vi "PDCDetectDrop.vi"(6 "Sensitivity [0-100]":dbl, 8 "Error In":errorcluster, 9 "RefImage":u16[](array[numeric]), 10 "CurrentImage":u16[](array[numeric]), 11 "DataDisplay":refnum<queue>) -> (0 "Error Out":errorcluster)   [LabVIEW 2015]
uses:
  TypeDefs/MessageCluster.ctl
  <vilib>/Analysis/NI_AALBase.lvlib
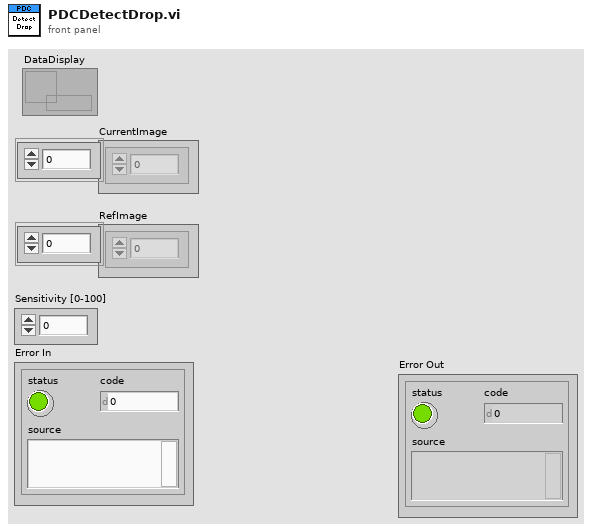
[diagram p1: front panel]
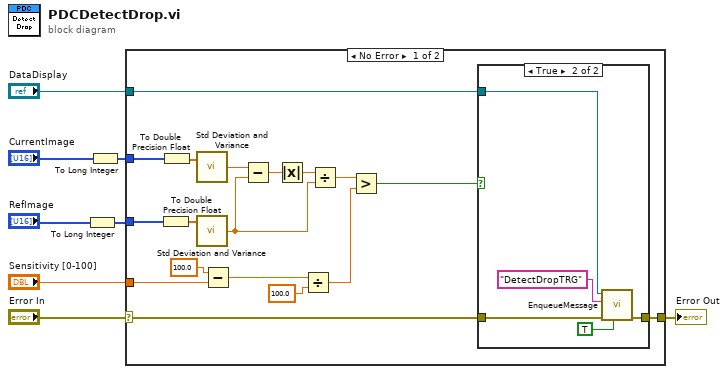
[diagram p0: block diagram]
diagram:
  n1 = To Long Integer(number="RefImage") -> (32bit integer=w4:i32[])
  n2 = To Long Integer(number="CurrentImage") -> (32bit integer=w2:i32[])
  n3 = case shown="No Error" "Error In" {
    selector: "Error In" -> [w25 w33]
    tunnel: [w26 w33] -> w7
    tunnel: "DataDisplay" -> [w24 _]
    tunnel: w4 -> [w22 _]
    tunnel: w2 -> [w23 _]
    tunnel: "Sensitivity [0-100]" -> [w10 _]
    frame No Error {
      n4 = To Double Precision Float(number=w22) -> (double precision float=w20:dbl[])
      n5 = To Double Precision Float(number=w23) -> (double precision float=w19:dbl[])
      n6 = call <vilib>:"Std Deviation and Variance.vi"("X"=w19) -> ("standard deviation"=w17:dbl)  [unwired: 1 in, 2 out]
      n7 = call <vilib>:"Std Deviation and Variance.vi"("X"=w20) -> ("standard deviation"=w14:dbl)  [unwired: 1 in, 2 out]
      n8 = Subtract(x=100.0, y=w10) -> (x-y=w9:dbl)
      n9 = Subtract(x=w17, y=w14) -> (x-y=w18:dbl)
      n10 = Absolute Value(x=w18) -> (abs(x)=w16:dbl)
      n11 = Divide(x=w9, y=100.0) -> (x/y=w11:dbl)
      n12 = Divide(x=w16, y=w14) -> (x/y=w15:dbl)
      n13 = Greater?(x=w15, y=w11) -> (0:w21:bool)
      n14 = case shown="True" w21 {
        tunnel: [w27 w32] -> w26
        tunnel: w25 -> [w27 w31]
        tunnel: w24 -> [_ w30]
        frame False {
        }
        frame True {
          n15 = call "EnqueueMessage.vi"("Priority Message? (F)"=TRUE, "error in (no error)"=w31, "Message"="DetectDropTRG", "MessageQueue"=w30) -> ("error out"=w32:errorcluster)  [unwired: 6 in, 1 out]
        }
      }
    }
    frame Error {
    }
  }
  "Error Out" <- w7
